vi "single_input_operation.vi"(1 "Operand":dbl, 2 "Operator":string(combo)) -> (0 "Result":dbl)   [LabVIEW 2018]
uses:
  <vilib>/gmath/NI_Gmath.lvlib
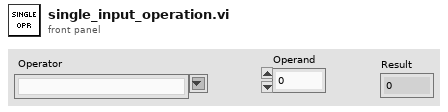
[diagram p1: front panel]
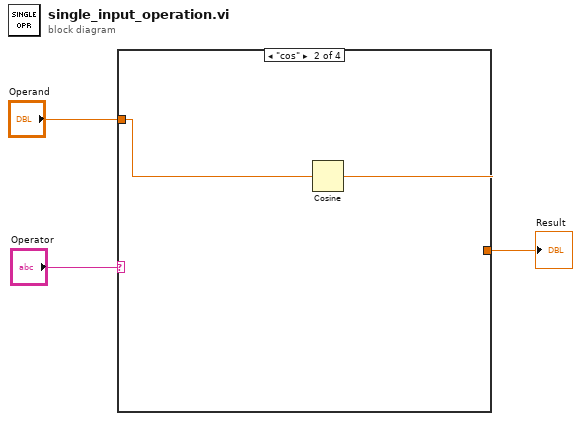
[diagram p0: block diagram]
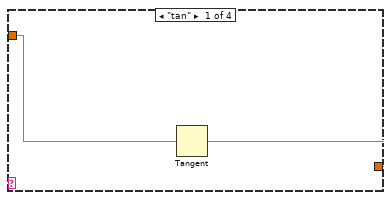
[diagram p2: hidden frame]
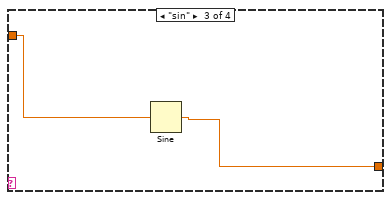
[diagram p3: hidden frame]
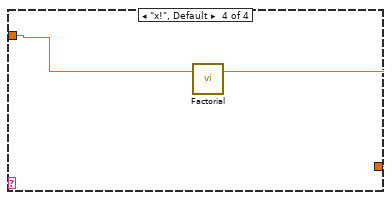
[diagram p4: hidden frame]
diagram:
  n1 = case shown="\"cos\"" "Operator" {
    tunnel: "Operand" -> [w5 w7 w9 w11]
    tunnel: [w4 w6 w8 w10] -> w1
    frame "tan" {
      n2 = Tangent(1:w5) -> (0:w4:dbl)
    }
    frame "cos" {
      n3 = Cosine(x=w7) -> (cos(x)=w6:dbl)
    }
    frame "sin" {
      n4 = Sine(x=w9) -> (sin(x)=w8:dbl)
    }
    frame "x!", Default {
      n5 = call <vilib>:"Factorial.vi"("n"=w11) -> ("n!"=w10:dbl)  [unwired: 2 in]
    }
  }
  "Result" <- w1
